vi "FINALNW.vi"(0 "L":bool, 1 "F":bool, 2 "Arduino Resource":T1, 3 "R":bool, 4 "Stop":bool, 7 "error in (no error)":errorcluster, 8 "B":bool) -> (10 "Boolean 3":bool, 12 "Boolean 1":bool, 14 "Boolean 4":bool, 15 "Voltage":dbl(knob) scale=0.0..5.0, 16 "error out 2":errorcluster, 17 "Arduino Resource out 2":T1, 18 "error out 3":errorcluster, 19 "Arduino Resource 4":T1, 20 "error out 4":errorcluster, 21 "Boolean out":bool, 22 "error out 6":errorcluster, 23 "Arduino Resource 2":T1, 24 "Arduino Resource 3":T1, 25 "Arduino Resource out":T1, 26 "Boolean 2":bool, 27 "error out":errorcluster)   [LabVIEW 2013]
uses:
  <vilib>/LabVIEW Interface for Arduino/Type Defs/Arduino Resource.ctl
  <vilib>/LabVIEW Interface for Arduino/Type Defs/Board Type.ctl
  <vilib>/LabVIEW Interface for Arduino/Type Defs/Analog Pin.ctl
  <vilib>/LabVIEW Interface for Arduino/LabVIEW Interface for Arduino.lvlib
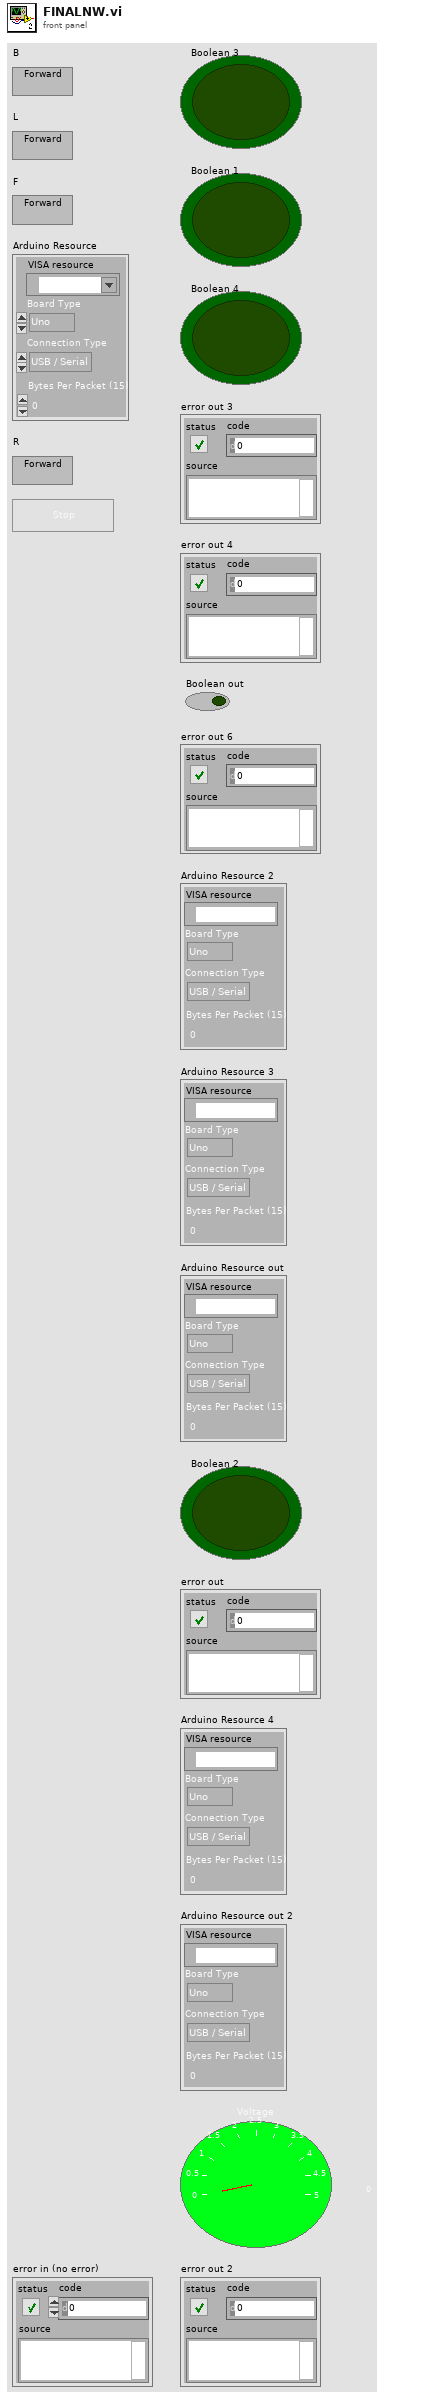
[diagram p1: front panel]
types:
  T1 = typedef "LabVIEW Interface for Arduino.lvlib/Arduino Resource.ctl" = cluster{"VISA resource":refnum<visa-resource-name>, "Board Type":T2, "Connection Type":enum8{"USB / Serial"}, "Bytes Per Packet (15)":u8}
  T2 = typedef "LabVIEW Interface for Arduino.lvlib/Board Type.ctl" = enum16{"Uno", "Dimuelanove w/Atmega 328", "Mega 2560"}
  T3 = typedef "LabVIEW Interface for Arduino.lvlib/Analog Pin.ctl" = enum8{"Anlog In 0", "Anlog In 1", "Anlog In 2", "Anlog In 3", "Anlog In 4", "Anlog In 5"}
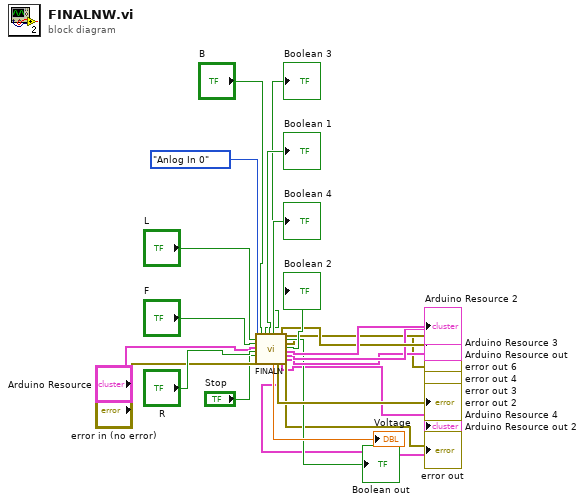
[diagram p0: block diagram]
diagram:
  n1 = call "FINALN.vi"("Analog Pin"=Analog_Pin."Anlog In 0", "L"="L", "F"="F", "Arduino Resource"="Arduino Resource", "R"="R", "Stop"="Stop", "error in (no error)"="error in (no error)", "B"="B") -> ("Boolean 3"=→"Boolean 3":bool, "Boolean 1"=→"Boolean 1":bool, "Boolean 4"=→"Boolean 4":bool, "Voltage"=→"Voltage":dbl, "error out 2"=→"error out 2":errorcluster, "Arduino Resource out 2"=→"Arduino Resource out 2":T1, "error out 3"=→"error out 3":errorcluster, "Arduino Resource 4"=→"Arduino Resource 4":T1, "error out 4"=→"error out 4":errorcluster, "Boolean out"=→"Boolean out":bool, "error out 6"=→"error out 6":errorcluster, "Boolean 2"=→"Boolean 2":bool, "Arduino Resource 2"=→"Arduino Resource 2":T1, "Arduino Resource 3"=→"Arduino Resource 3":T1, "Arduino Resource out"=→"Arduino Resource out":T1, "error out"=→"error out":errorcluster)  [unwired: 4 in]
